vi "RSZVB Get Port Configuration.vi"(8 "error in (no error)":errorcluster {"code" format="%.0x"}, 10 "Channel (1)":i32=1, 11 "VISA session":refnum<visa-resource-name>) -> (0 "error out":errorcluster {"code" format="%.0x"}, 1 "Port Group B":i32, 2 "Port Group A":i32, 3 "dup VISA session":refnum<visa-resource-name>, 4 "Port Group D":i32, 5 "Port Group C":i32)   [LabVIEW 2011]
doc: "This VI returns the internal signal paths of the multiport test set R&S ZV-Z83 for channel no. <Ch>. \n\nRemote-control command(s):\nROUTe<Ch>:PORTs?"
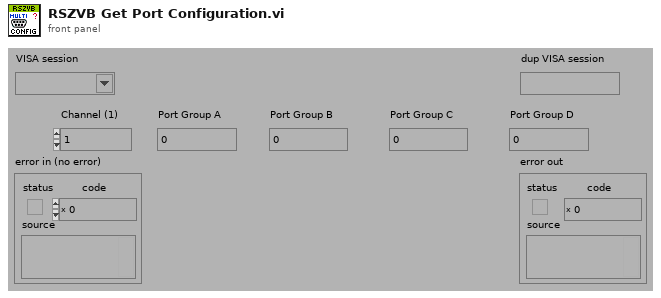
[diagram p1: front panel]
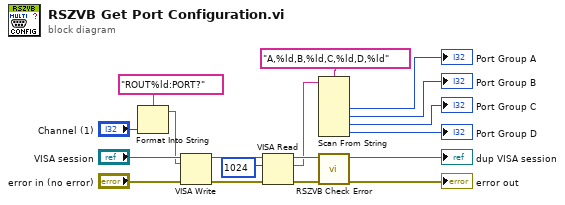
[diagram p0: block diagram]
diagram:
  n1 = Format Into String(format string="ROUT%ld:PORT?", "Channel (1)") -> (resulting string=w8:string)  [unwired: 2 in, 1 out]
  n2 = VISA Write(VISA resource name="VISA session", write buffer=w8, error in (no error)="error in (no error)") -> (VISA resource name out=w18:refnum<visa-resource-name>, error out=w17:errorcluster)  [unwired: 1 out]
  n3 = VISA Read(VISA resource name=w18, byte count=u32 1024 ("byte count (0)"), error in (no error)=w17) -> (VISA resource name out=w15:refnum<visa-resource-name>, read buffer=w1:string, error out=w14:errorcluster)  [unwired: 1 out]
  n4 = Scan From String(format string="A,%ld,B,%ld,C,%ld,D,%ld", input string=w1) -> (output 1=→"Port Group A":i32, output 2=→"Port Group B":i32, output 3=→"Port Group C":i32, output 4=→"Port Group D":i32)  [unwired: 6 in, 3 out]
  n5 = call "RSZVB Check Error.vi"("error in (no error)"=w14, "VISA session"=w15) -> ("error out"=→"error out":errorcluster, "dup VISA session"=→"dup VISA session":refnum<visa-resource-name>)  [unwired: 8 in]
